vi "cornell-K0s.vi"(6 "Numeric":i32=500, 10 "s":dbl, 11 "ω":dbl) -> (0 "Ks(ω)":cdb)   [LabVIEW 2020]
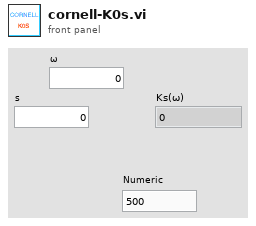
[diagram p1: front panel]
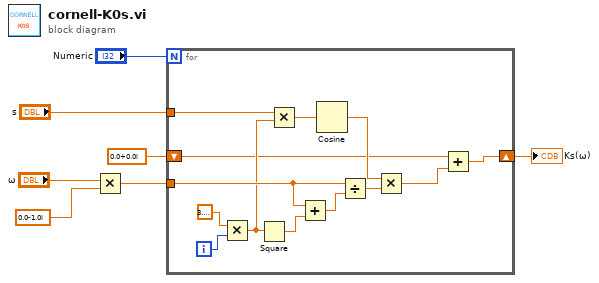
[diagram p0: block diagram]
diagram:
  n1 = Multiply(x="ω", y=cdb 0.0-1.0i ("x")) -> (x*y=w6:cdb)
  n2 = for {
    N: "Numeric" -> [_]
    tunnel: w6 -> [w17]
    tunnel: "s" -> [w15]
    shift-right: [w8] -> w4
    shift-left: cdb 0.0+0.0i ("x") -> [w10]
    i -> [w19]
    n3 = Multiply(x=3.141592653589793, y=w19) -> (x*y=w14:dbl)
    n4 = Square(x=w14) -> (x^2=w18:dbl)
    n5 = Multiply(x=w15, y=w14) -> (x*y=w13:dbl)
    n6 = Add(x=w17, y=w18) -> (x+y=w16:cdb)
    n7 = Cosine(x=w13) -> (cos(x)=w12:dbl)
    n8 = Divide(x=w17, y=w16) -> (x/y=w11:cdb)
    n9 = Multiply(x=w12, y=w11) -> (x*y=w9:cdb)
    n10 = Add(x=w10, y=w9) -> (x+y=w8:cdb)
  }
  "Ks(ω)" <- w4
